vi "Group by Parent.vi"(11 "List of Runnables":string[](array[string])) -> (3 "Methods":cluster{"Methods":string[]}[](array[cluster]))   [LabVIEW 2020, in "Parallel Test Runner.lvclass"]
uses:
  Parallel Test Runner.lvclass
  <vilib>/Utility/miscctls.llb/LVMapReplaceAction.ctl
panel:
  out "map":map{string, string[]}(c390)
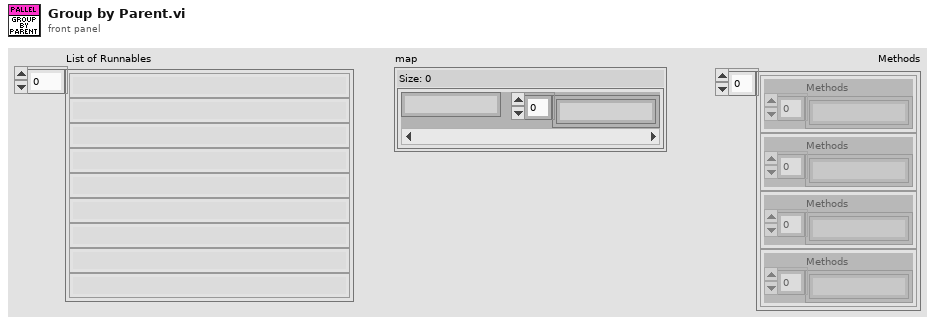
[diagram p1: front panel]
types:
  T1 = typedef "LVMapReplaceAction.ctl" = enum32{"Modify Entry only if found", "Add or Modify Entry", "Delete Entry"}
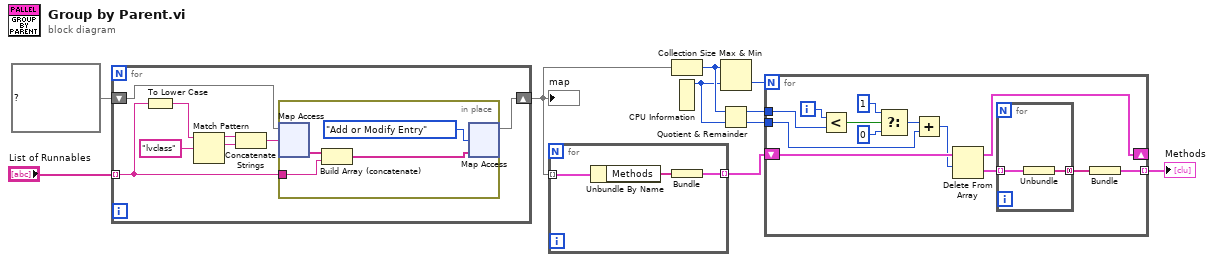
[diagram p0: block diagram]
diagram:
  n1 = for {
    tunnel: "List of Runnables" -> [w13] mode=indexing
    shift-right: [w17] -> w8
    shift-left: map{string, string[]} {} ("map") -> [w18]
    n2 = To Lower Case(string=w13) -> (all lower case string=w11:string)
    n3 = Match Pattern(string=w11, regular expression="lvclass") -> (before substring=w15:string, match substring=w14:string)  [unwired: 1 in, 2 out]
    n4 = Concatenate Strings(w15, w14) -> (w12:string)
    n5 = in-place {
      in-place-border: w13 -> [w20]
      n6 = in-place-map #1(w18, w12) -> (w22:string[])  [unwired: 1 in, 1 out]
      n7 = Build Array (concatenate)(w22, w20) -> (w21:string[])
      n8 = in-place-map #1(w21, LVMapReplaceAction."Add or Modify Entry" ("action")) -> (w17:map{string, string[]})  [unwired: 2 out]
    }
  }
  "map" <- w8
  n9 = for {
    tunnel: w8 -> [w25] mode=indexing
    tunnel: [w23] -> w4 mode=indexing
    n10 = Unbundle By Name(w25) -> ("Methods"=w24:string[])
    n11 = Bundle("Methods"=w24) -> (w23:cluster{"Methods":string[]})  [unwired: 1 in]
  }
  n12 = Collection Size(1:w8) -> (0:w3:i32)
  n13 = CPU Information() -> (4:w2:i32)  [unwired: 3 out]
  n14 = Max & Min(x=w3, y=w2) -> (min(x,y)=w1:i32)  [unwired: 1 out]
  n15 = Quotient & Remainder(x=w3, y=w2) -> (x-y*floor(x/y)=w7:i32, floor(x/y)=w6:i32)
  n16 = for {
    N: w1 -> [_]
    tunnel: [w33] -> w5 mode=indexing
    tunnel: w7 -> [w37]
    tunnel: w6 -> [w35]
    shift-right: [w26] -> _
    shift-left: w4 -> [w38]
    i -> [w36]
    n17 = Less?(x=w36, y=w37) -> (x < y?=w32:bool)
    n18 = Select(t=1 ("x*y"), s=w32, f=0 ("x*y")) -> (s? t:f=w31:i32)
    n19 = Add(x=w31, y=w35) -> (x+y=w28:i32)
    n20 = Delete From Array(array=w38, length=w28) -> (deleted portion=w27:cluster{"Methods":string[]}[], array with subset deleted=w26:cluster{"Methods":string[]}[])  [unwired: 1 in]
    n21 = for {
      tunnel: w27 -> [w40] mode=indexing
      tunnel: [w39] -> w34 mode=concatenating
      n22 = Unbundle(w40) -> ("Methods"=w39:string[])
    }
    n23 = Bundle("Methods"=w34) -> (w33:cluster{"Methods":string[]})  [unwired: 1 in]
  }
  "Methods" <- w5
